vi "数据格式转化.vi"() -> ()   [LabVIEW 2021]
uses:
  <vilib>/Utility/file.llb/Write Delimited Spreadsheet (DBL).vi
panel:
  out "错误输出":errorcluster
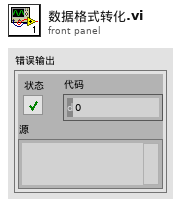
[diagram p1: front panel]
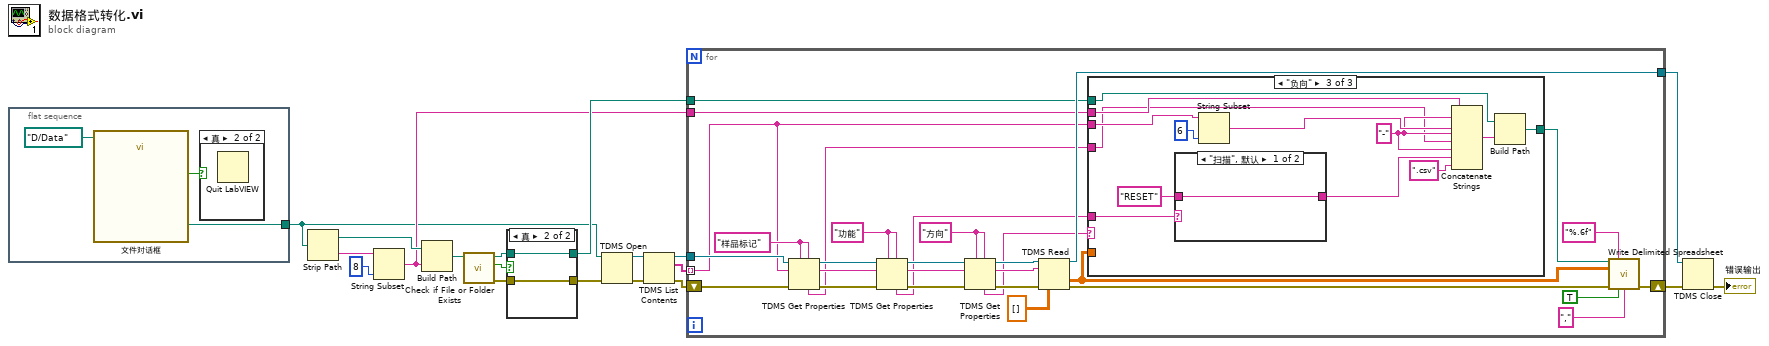
[diagram p0: block diagram]
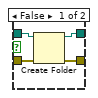
[diagram p3: hidden frame]
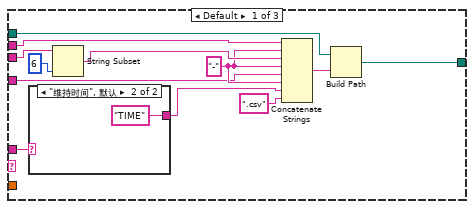
[diagram p4: hidden frame]
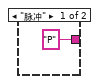
[diagram p5: hidden frame]
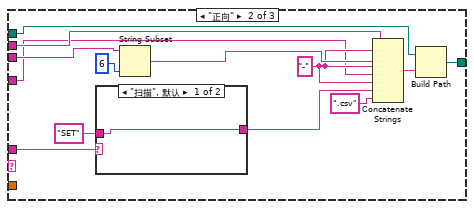
[diagram p6: hidden frame]
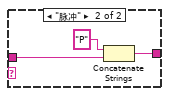
[diagram p7: hidden frame]
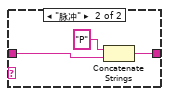
[diagram p8: hidden frame]
diagram:
  n1 = flat-sequence {
    tunnel: [w21] -> w1
    frame #0 {
      n2 = call "文件对话框"("start path"=path "D:/Data") -> ("selected path"=w21:path, "cancelled"=w20:bool)  [unwired: 11 in, 2 out]
      n3 = case shown="真" w20 {
        frame False {
        }
        frame True {
          n4 = Quit LabVIEW() -> ()  [unwired: 1 in]
        }
      }
    }
  }
  n5 = Strip Path(path=w1) -> (stripped path=w14:path, name=w16:string)
  n6 = String Subset(string=w16, length (rest)=8 ("长度（剩余）")) -> (substring=w9:string)  [unwired: 1 in]
  n7 = Build Path(base path=w14, name or relative path=w9) -> (appended path=w13:path)
  n8 = call <vilib>:"Check if File or Folder Exists.vi"("path"=w13) -> ("error out"=w7:errorcluster, "file or folder exists?"=w12:bool, "dup path"=w11:path)  [unwired: 8 in]
  n9 = case shown="真" w12 {
    tunnel: w11 -> [w26 w28]
    tunnel: [w25 w28] -> w10
    tunnel: w7 -> [w24 w27]
    tunnel: [w23 w27] -> w6
    frame False {
      n10 = Create Folder(path (use dialog)=w26, error in=w24) -> (created path=w25:path, error out=w23:errorcluster)  [unwired: 1 in, 1 out]
    }
    frame True {
    }
  }
  n11 = TDMS Open(8:w6, 11:w1) -> (0:w5:errorcluster, 3:w19:refnum<k34>)  [unwired: 5 in]
  n12 = TDMS List Contents(4:w5, 7:w19) -> (0:w4:errorcluster, 2:w18:string[], 3:w17:refnum<k34>)  [unwired: 1 in, 1 out]
  n13 = for {
    tunnel: w18 -> [w36] mode=indexing
    tunnel: w17 -> [w57]
    tunnel: w10 -> [w39]
    tunnel: w9 -> [w35]
    tunnel: [w46] -> w8
    shift-right: [w29] -> w3
    shift-left: w4 -> [w45]
    w47 = "方向" ("属性名称")
    w49 = "样品标记" ("属性名称")
    w48 = "功能" ("属性名称")
    n14 = TDMS Get Properties(5:w49, 7:w49, 8:w45, 10:w36, 11:w57) -> (0:w44:errorcluster, 2:w55:string, 3:w56:refnum<k34>, 4:w34:string)  [unwired: 1 in, 2 out]
    n15 = TDMS Get Properties(5:w48, 7:w48, 8:w44, 10:w55, 11:w56) -> (0:w43:errorcluster, 2:w53:string, 3:w54:refnum<k34>, 4:w37:string)  [unwired: 1 in, 2 out]
    n16 = TDMS Get Properties(5:w47, 7:w47, 8:w43, 10:w53, 11:w54) -> (0:w42:errorcluster, 2:w52:string, 3:w51:refnum<k34>, 4:w38:string)  [unwired: 1 in, 2 out]
    n17 = TDMS Read(0:w51, 5:w52, 11:w42, 12:dbl[][] []) -> (4:w46:refnum<k34>, 10:w41:dbl[][], 15:w40:errorcluster)  [unwired: 4 in, 3 out]
    n18 = case shown="\"负向\"" w38 {
      tunnel: w41 -> [_ _ _]
      tunnel: w39 -> [w66 w81 w98]
      tunnel: w37 -> [w65 w80 w97]
      tunnel: w36 -> [w63 w78 w95]
      tunnel: w35 -> [w62 w77 w94]
      tunnel: w34 -> [w60 w75 w92]
      tunnel: [w58 w72 w89] -> w33
      frame Default {
        w61 = "-" ("字符串")
        n19 = case shown="\"维持时间\", 默认" w65 {
          tunnel: ["P" ("字符串") "TIME" ("f")] -> w68
          frame "脉冲" {
          }
          frame "维持时间", Default {
          }
        }
        n20 = String Subset(string=w63, length (rest)=6 ("长度（剩余）")) -> (substring=w67:string)  [unwired: 1 in]
        n21 = Concatenate Strings(w62, w61, w67, w61, w60, w61, w68, ".csv" ("字符串")) -> (w69:string)
        n22 = Build Path(base path=w66, name or relative path=w69) -> (appended path=w58:path)
      }
      frame "正向" {
        w76 = "-" ("字符串")
        n23 = case shown="\"扫描\", 默认" w80 {
          tunnel: "SET" ("t") -> [w85 w88]
          tunnel: [w85 w86] -> w83
          frame "扫描", Default {
          }
          frame "脉冲" {
            n24 = Concatenate Strings("P" ("字符串"), w88) -> (w86:string)
          }
        }
        n25 = String Subset(string=w78, length (rest)=6 ("长度（剩余）")) -> (substring=w82:string)  [unwired: 1 in]
        n26 = Concatenate Strings(w77, w76, w82, w76, w75, w76, w83, ".csv" ("字符串")) -> (w84:string)
        n27 = Build Path(base path=w81, name or relative path=w84) -> (appended path=w72:path)
      }
      frame "负向" {
        w93 = "-" ("字符串")
        n28 = case shown="\"扫描\", 默认" w97 {
          tunnel: "RESET" ("f") -> [w102 w105]
          tunnel: [w102 w103] -> w100
          frame "扫描", Default {
          }
          frame "脉冲" {
            n29 = Concatenate Strings("P" ("字符串"), w105) -> (w103:string)
          }
        }
        n30 = String Subset(string=w95, length (rest)=6 ("长度（剩余）")) -> (substring=w99:string)  [unwired: 1 in]
        n31 = Concatenate Strings(w94, w93, w99, w93, w92, w93, w100, ".csv" ("字符串")) -> (w101:string)
        n32 = Build Path(base path=w98, name or relative path=w101) -> (appended path=w89:path)
      }
    }
    n33 = call-poly <vilib>:"Write Delimited Spreadsheet.vi"("file path (dialog if empty)"=w33, "format (%.3f)"="%.6f", "2D data"=w41, "error in (no error)"=w40, "transpose? (no:F)"=TRUE, "delimiter (\\t)"="," ("delimiter (\\t)")) -> ("error out"=w29:errorcluster)  [unwired: 8 in, 1 out]
  }
  n34 = TDMS Close(8:w3, 11:w8) -> (0:→"错误输出":errorcluster)  [unwired: 1 out]
